vi "DesktopAppSettingsFGV.vi"(8 "FGVAction (Read)":T7, 11 "DesktopAppSettingsIn":T1={"MobileAnalyzer IP"="//172.22.11.2", "Network Stream Timeout Code"=-314004, "Endpoint Destroyed Code"=0, "Save to file?"=FALSE, "All threads"=[], "Connected"=FALSE, "SaveSignalsDir"=path "1234", "SaveAnalysisOnPC?"=FALSE, "AnalysisSettings"={"Fault Thresholds"={"Parameters labels"=[], "Parameters thresholds"=[], "Freqs and thresholds"=[], "Orders and thresholds"=[]}, "Analysis series name"="Analiza", "Save data analysis?"=TRUE, "F-Band Size"=20, "OrderAnalysis?"=TRUE, "Accelerometer"=enum."MMA7351", "fs [Hz]"=4000.0, "Pulse per revolution"=1, "FFT-Parameters"={"averaging mode"=enum."No averaging", "weighting mode"=enum."Linear", "number of averages"=0}, "O-WindowPowerSpectrum"=0, "O-SpectrumAveraging"=enum."No averaging", "O-MaxOrder"=0.0, "O-Resolution"=0.0, "O-BandSize"=0.0, "FrameLength [s]"=1.0, "Aq.FrameLength [ms]"=0, "FilterOrder"=0, "Sensitivity [V/g]"=[]}}) -> (3 "DesktopAppSettingsOut":T1={"MobileAnalyzer IP"="//172.22.11.2", "Network Stream Timeout Code"=-314004, "Endpoint Destroyed Code"=0, "Save to file?"=FALSE, "All threads"=[], "Connected"=FALSE, "SaveSignalsDir"=path "1234", "SaveAnalysisOnPC?"=FALSE, "AnalysisSettings"={"Fault Thresholds"={"Parameters labels"=[], "Parameters thresholds"=[], "Freqs and thresholds"=[], "Orders and thresholds"=[]}, "Analysis series name"="Analiza", "Save data analysis?"=TRUE, "F-Band Size"=20, "OrderAnalysis?"=TRUE, "Accelerometer"=enum."MMA7351", "fs [Hz]"=4000.0, "Pulse per revolution"=1, "FFT-Parameters"={"averaging mode"=enum."No averaging", "weighting mode"=enum."Linear", "number of averages"=0}, "O-WindowPowerSpectrum"=0, "O-SpectrumAveraging"=enum."No averaging", "O-MaxOrder"=0.0, "O-Resolution"=0.0, "O-BandSize"=0.0, "FrameLength [s]"=1.0, "Aq.FrameLength [ms]"=0, "FilterOrder"=0, "Sensitivity [V/g]"=[]}})   [LabVIEW 2019]
uses:
  MobileAnalyzer/mainVIs/utilities/FGVAction.ctl
  DesktopAppSettings.ctl
  masterVIs/Thread.ctl
  DialogsVIs/AnalysisSettings.ctl
  MobileAnalyzer/mainVIs/analyzeAccelerationDataVIs/calculateFaultIndicatorsVIs/Thresholds.ctl
  MobileAnalyzer/mainVIs/analyzeAccelerationDataVIs/calculateFaultIndicatorsVIs/FaultParameter.ctl
  MobileAnalyzer/mainVIs/aquireAccelerationDataVIs/Accelerometer.ctl
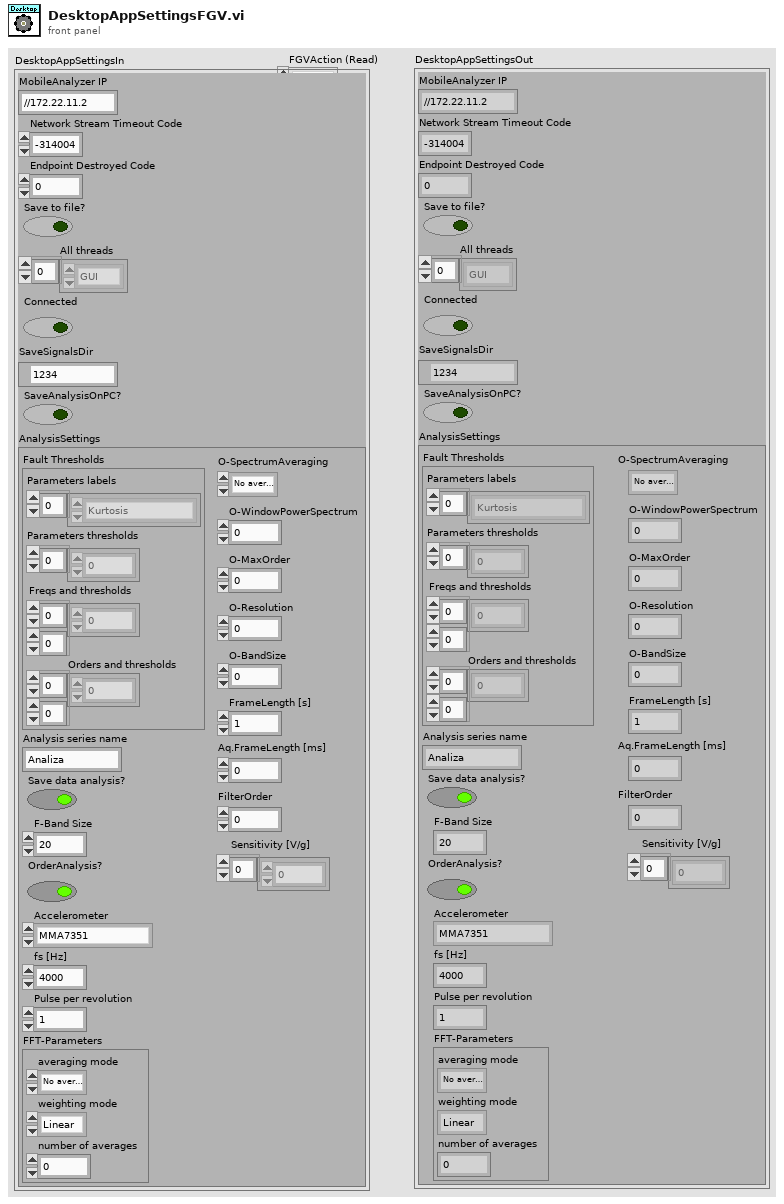
[diagram p1: front panel]
types:
  T1 = typedef "DesktopAppSettings.ctl" = cluster{"MobileAnalyzer IP":string, "Network Stream Timeout Code":i32, "Endpoint Destroyed Code":i32, "Save to file?":bool, "All threads":T2[], "Connected":bool, "SaveSignalsDir":path, "SaveAnalysisOnPC?":bool, "AnalysisSettings":T3}
  T2 = typedef "Thread.ctl" = enum16{"GUI", "communicateWithAnalyzer", "saveDataToTDMS"}
  T3 = typedef "AnalysisSettings.ctl" = cluster{"Fault Thresholds":T4, "Analysis series name":string, "Save data analysis?":bool, "F-Band Size":i32, "OrderAnalysis?":bool, "Accelerometer":T6, "fs [Hz]":dbl, "Pulse per revolution":u16, "FFT-Parameters":cluster{"averaging mode":enum16{"No averaging", "Vector averaging", "RMS averaging", "Peak hold"}, "weighting mode":enum16{"Linear", "Exponential"}, "number of averages":u32}, "O-WindowPowerSpectrum":u32, "O-SpectrumAveraging":enum16{"No averaging", "Vector averaging", "RMS averaging", "Peak hold"}, "O-MaxOrder":dbl, "O-Resolution":dbl, "O-BandSize":dbl, "FrameLength [s]":dbl, "Aq.FrameLength [ms]":i64, "FilterOrder":i32, "Sensitivity [V/g]":dbl[]}
  T4 = typedef "Thresholds.ctl" = cluster{"Parameters labels":T5[], "Parameters thresholds":dbl[], "Freqs and thresholds":dbl[][], "Orders and thresholds":dbl[][]}
  T5 = typedef "FaultParameter.ctl" = enum16{"Kurtosis", "RMS", "Crest factor"}
  T6 = typedef "Accelerometer.ctl" = enum16{"None", "MPU6050", "MMA7351"}
  T7 = typedef "FGVAction.ctl" = enum16{"Read", "Write"}
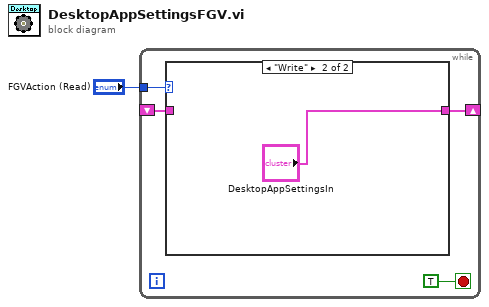
[diagram p0: block diagram]
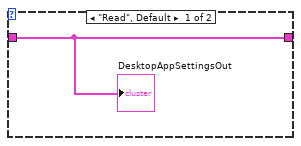
[diagram p2: hidden frame]
diagram:
  n1 = while {
    tunnel: "FGVAction (Read)" -> [w4]
    shift-right: [w2] -> _
    shift-left: _ -> [w3]
    stop <- TRUE stop-if-true
    n2 = case shown="\"Write\"" w4 {
      tunnel: w3 -> [w6 _]
      tunnel: [w6 "DesktopAppSettingsIn"] -> w2
      frame "Read", Default {
        "DesktopAppSettingsOut" <- w6
      }
      frame "Write" {
      }
    }
  }
